vi "sbRIO-9651.DAC Example.RT Main.vi"() -> ()   [LabVIEW 2015]
doc: "This example is based on the MAX5216. It allows you to control the voltage output on the SPI chip. This VI interfaces with the SPI Engine on the FPGA."
uses:
  <vilib>/userdefined/High Color/nirio_resource_hc.ctl
  <vilib>/FPGAPlugInAG/sbRIO-9651/niLvFpga_Open_sbRIO-9651.vi
  <vilib>/rvi/interface/common/dynamic/niFpgaDynamicAddResources.vi
  <vilib>/FPGAPlugInAG/Dynamic/niLvFpga_Reset_Dynamic.vi
  <vilib>/FPGAPlugInAG/Dynamic/niLvFpga_Run_Dynamic.vi
  <vilib>/Utility/error.llb/Error Cluster From Error Code.vi
  <vilib>/rvi/errors/niLvFpgaAdjustHostInterfaceError.vi
  <vilib>/FPGAPlugInAG/Dynamic/niLvFpga_Close_Dynamic.vi
  <vilib>/rvi/interface/nirviOpenFPGA/nirviOpenFPGA.xnode
  FPGA Bitfiles/SPIAPI-sbRIO-965_FPGATarget_sbRIO-9651.DACEx_zE1viy5ZTkI.lvbitx
  <vilib>/rvi/interface/nirviMethod/nirviMethod.xnode
  <vilib>/rvi/interface/nirviReadWriteControl/nirviReadWriteControl.xnode
  <vilib>/rvi/interface/nirviCloseFPGA/nirviCloseFPGA.xnode
  <vilib>/rvi/interface/Simulation/niFpgaSimulationCallBeginRW.vi
  NiFpgaLv.dll
panel:
  in  "SPI Engine Clock Divisor":u8
  in  "Transfer Length (bits)":u8=32
  in  "FPGA Resource":T1="RIO0"
  in  "Reference Voltage":dbl=3.0 format="%f"
  out "Binary to DAC":u64 format="%024b"
  in  "Voltage Output":dbl=3.0 format="%f"
  in  "Sample Rate (S/s)":u32=10
  in  "stop":bool
  # "SPI Settings"
  # "Overview: This example is based on the MAX5216.  It allows you to control the\nvoltage output on the SPI chip. \nRequirements: LabVIEW Full Development System, LabVIEW Real Time, \nLabVIEW FPGA, MAX5216, NI System on Module, NI 9651.\nInstructions:\n1. The SPI PHY Settings are already setup for the MAX5216.  Do not adjust them.\n2. Plug the MAX5216 into PMOD1 on the NI 9651.\n3. Setup Vref according to the user manual.\n4. Run the VI.\n5. Adjust the Voltage Output and observe the voltage change on the MAX5216."
  # "120 MHz Engine Clock / 42 =\n2.85 MHz SCLK"
  # "DAC Settings"
  # "MSB"
  # "LSB"
  # "This example is based on the MAX5216.  The datasheets for this particular device are available here:\nhttp://datasheets.maximintegrated.com/en/ds/MAX5214-MAX5216.pdf\nhttp://datasheets.maximintegrated.com/en/ds/MAX5216PMB1.pdf"
  # "Sampling Info"
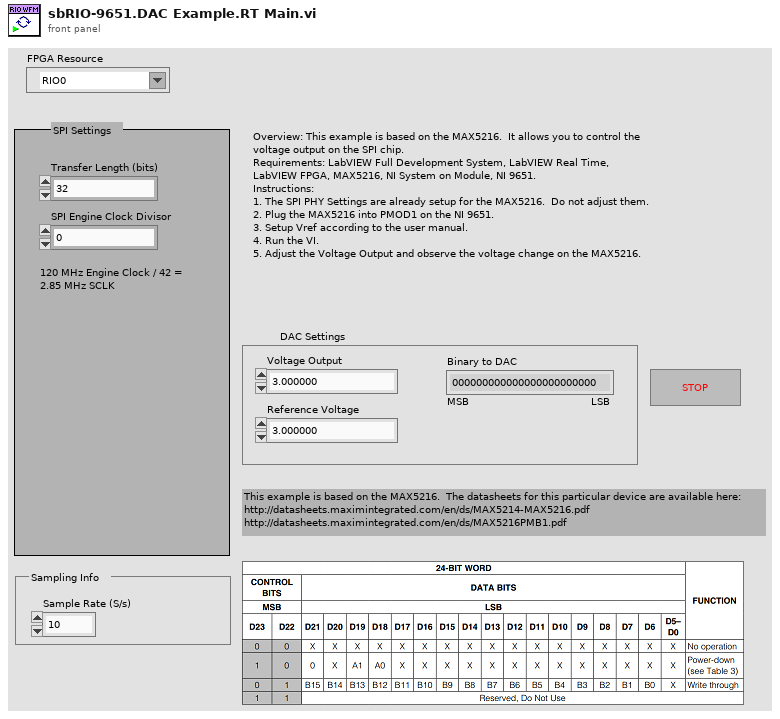
[diagram p1: front panel]
types:
  T1 = typedef "nirio_resource_hc.ctl" = tag
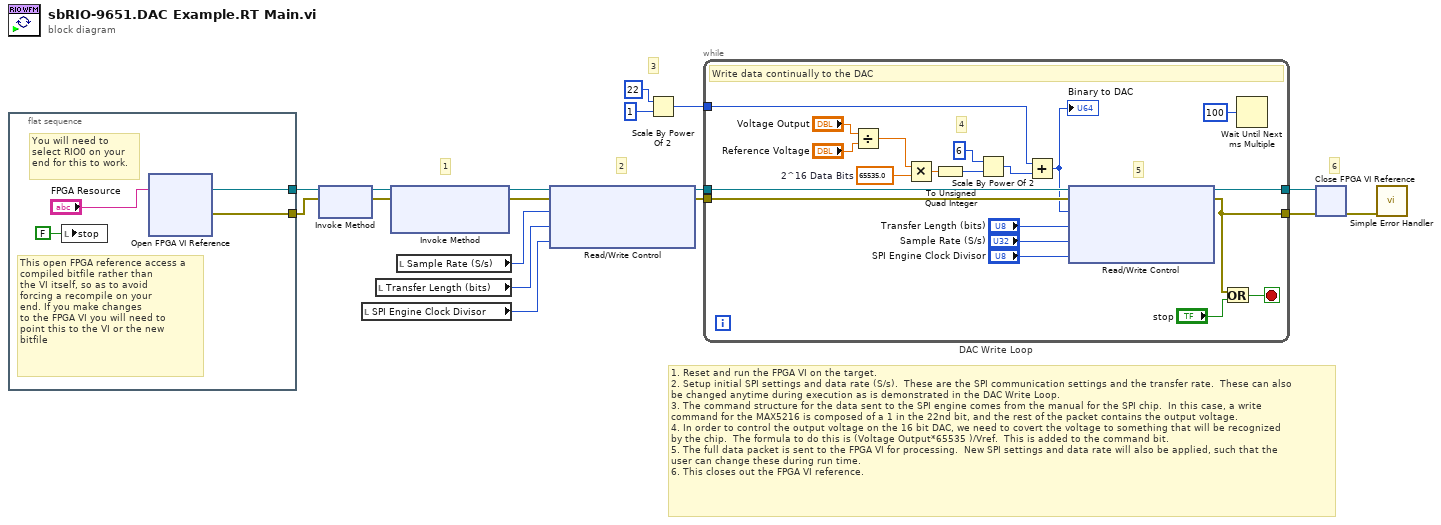
[diagram p0: block diagram]
diagram:
  # "1. Reset and run the FPGA VI on the target.\n2. Setup initial SPI settings and data rate (S/s).  These are the SPI communication settings and the transfer rate.  These can also\nbe changed anytime during execution as is demonstrated in the DAC Write Loop.\n3. The command structure for the data sent to the SPI engine comes from the manual for the SPI chip.  In this case, a write\ncommand for the MAX5216 is composed of a 1 in the 22nd bit, and the rest of the packet contains the output voltage.\n4. In order to control the output voltage on the 16 bit DAC, we need to covert the voltage to something that will be recognized\nby the chip.  The formula to do this is (Voltage Output*65535 )/Vref.  This is added to the command bit.\n5. The full data packet is sent to the FPGA VI for processing.  New SPI settings and data rate will also be applied, such that the\nuser can change these during run time.\n6. This closes out the FPGA VI reference."
  # "6"
  # "3"
  # "2"
  # "1"
  n1 = flat-sequence {
    tunnel: [w20] -> w17
    tunnel: [w19] -> w16
    frame #0 {
      # "You will need to\nselect RIO0 on your\nend for this to work."
      # "This open FPGA reference access a\ncompiled bitfile rather than \nthe VI itself, so as to avoid\nforcing a recompile on your\nend. If you make changes\nto the FPGA VI you will need to\npoint this to the VI or the new\nbitfile"
      n2 = local write "stop"(FALSE ("stop")) -> ()
      n3 = xnode "Open FPGA VI Reference"("resource name"="FPGA Resource") -> ("FPGA VI Reference Out"=w20:refnum<k20>, "error out"=w19:errorcluster)  [unwired: 1 in]
    }
  }
  n4 = xnode "Invoke Method"("FPGA VI Reference In"=w17, "error in"=w16) -> ("FPGA VI Reference Out"=w11:refnum<k20>, "error out"=w10:errorcluster)
  n5 = local read "SPI Engine Clock Divisor"() -> (w1:u8)
  n6 = local read "Transfer Length (bits)"() -> (w2:u8)
  n7 = xnode "Invoke Method"("FPGA VI Reference In"=w11, "error in"=w10) -> ("FPGA VI Reference Out"=w12:refnum<k20>, "error out"=w14:errorcluster)  [unwired: 1 in]
  n8 = local read "Sample Rate (S/s)"() -> (w3:u32)
  n9 = xnode "Read/Write Control"("FPGA VI Reference In"=w12, "error in"=w14, "Sample Rate (S/s)"=w3, "Transfer Length (bits)"=w2, "SPI Engine Clock Divisor"=w1) -> ("FPGA VI Reference Out"=w9:refnum<k20>, "error out"=w13:errorcluster)
  n10 = Scale By Power Of 2(n=i16 22, x=u64 1) -> (x*2^n=w6:u64)
  n11 = while "DAC Write Loop" {
    tunnel: w9 -> [w39]
    tunnel: w13 -> [w38]
    tunnel: w6 -> [w25]
    tunnel: [w37] -> w5
    tunnel: [w24] -> w4
    stop <- w41 stop-if-true
    w32 = 65535.0  # 2^16 Data Bits
    # "4"
    # "5"
    # "Write data continually to the DAC"
    n12 = Divide(x="Voltage Output", y="Reference Voltage") -> (x/y=w31:dbl)
    n13 = Multiply(x=w31, y=w32) -> (x*y=w30:dbl)
    n14 = To Unsigned Quad Integer(1:w30) -> (0:w29:u64)
    n15 = Scale By Power Of 2(n=i16 6, x=w29) -> (x*2^n=w27:u64)
    n16 = Add(x=w25, y=w27) -> (x+y=w26:u64)
    "Binary to DAC" <- w26
    n17 = xnode "Read/Write Control"("FPGA VI Reference In"=w39, "error in"=w38, "Data To Write"=w26, "Transfer Length (bits)"="Transfer Length (bits)", "Sample Rate (S/s)"="Sample Rate (S/s)", "SPI Engine Clock Divisor"="SPI Engine Clock Divisor") -> ("FPGA VI Reference Out"=w37:refnum<k20>, "error out"=w24:errorcluster)
    n18 = Or(x=w24, y="stop") -> (x .or. y?=w41:bool)
    n19 = Wait Until Next ms Multiple(millisecond multiple=u32 100 ("milliseconds to wait")) -> ()  [unwired: 1 out]
  }
  n20 = xnode "Close FPGA VI Reference"("FPGA VI Reference In"=w5, "error in"=w4) -> ("error out"=w15:errorcluster)
  n21 = call <vilib>:"Simple Error Handler.vi"("error in (no error)"=w15) -> ()  [unwired: 1 in, 8 out]
